vi "进度条.vi"() -> ()   [LabVIEW 2018]
panel:
  in  "诊断结果显示":bool
  out "水平刻度条":dbl(slide) scale=0.0..100.0
  out "进度显示":dbl format="%#.2f%%"
  # "病症诊断进度："
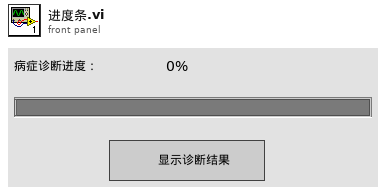
[diagram p1: front panel]
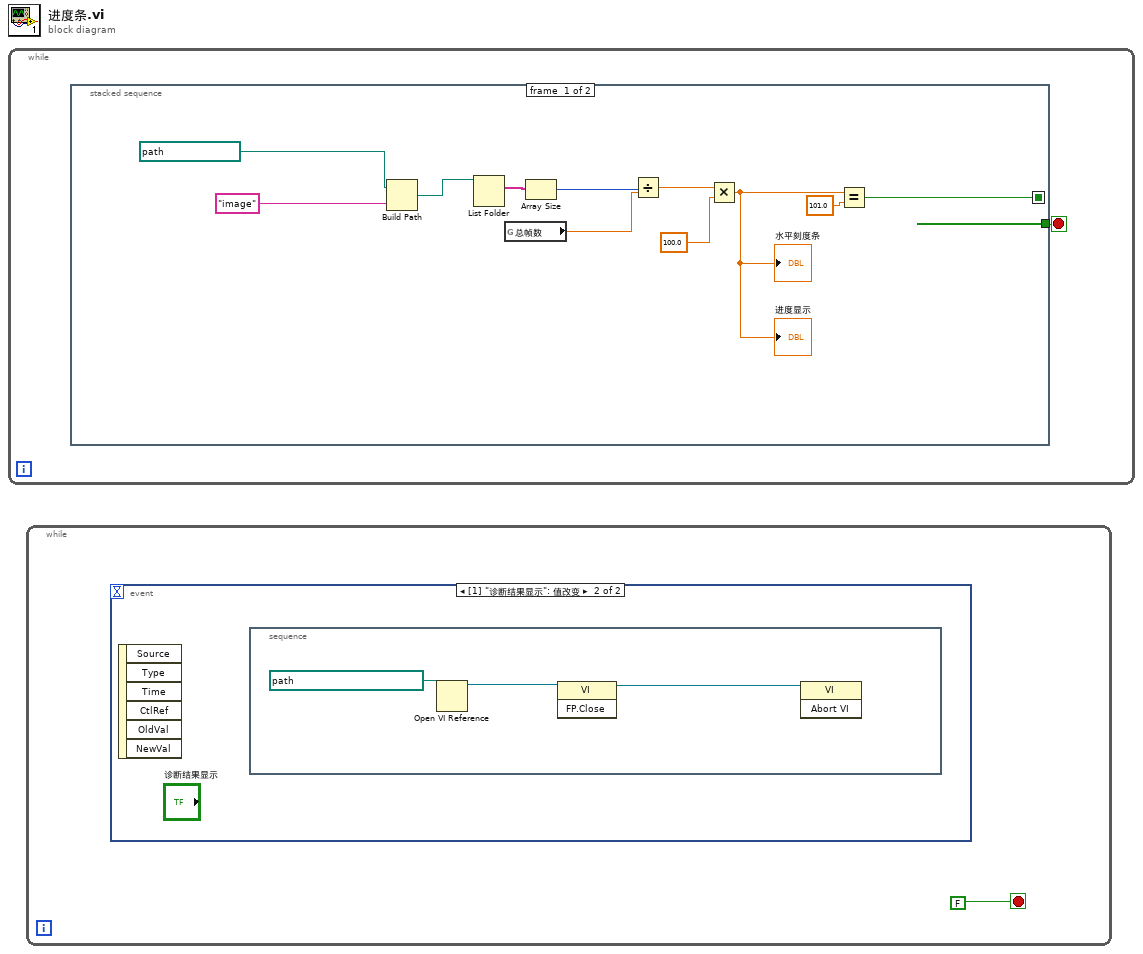
[diagram p0: block diagram]
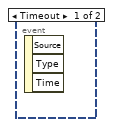
[diagram p2: hidden frame]
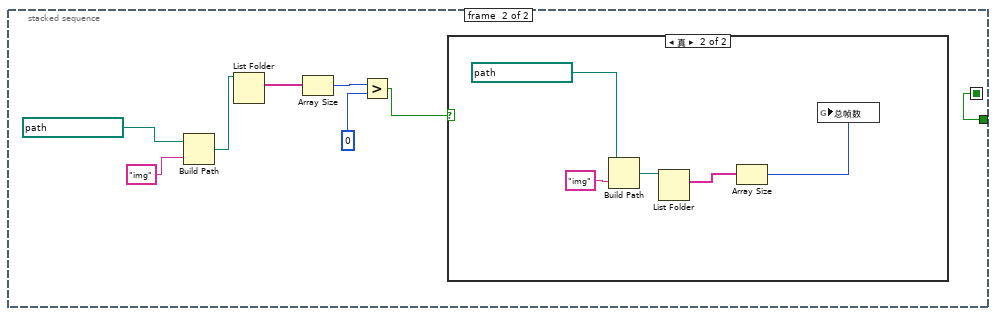
[diagram p3: hidden frame]
diagram:
  n1 = while {
    stop <- w1 stop-if-true
    n2 = stacked-sequence {
      seq-local: [w5 _] -> [_ w20]
      tunnel: [_ w20] -> w1
      frame #0 {
        n3 = Build Path(base path=path "E:/登陆系统重写", name or relative path="image" ("名称或相对路径")) -> (appended path=w10:path)
        n4 = List Folder(path=w10) -> (filenames=w11:string[])  [unwired: 3 in, 3 out]
        n5 = global read "全局变量.vi" "总帧数"() -> (w4:dbl)
        n6 = Array Size(array=w11) -> (size(s)=w3:i32)
        n7 = Divide(x=w3, y=w4) -> (x/y=w8:dbl)
        n8 = Multiply(x=w8, y=100.0) -> (x*y=w7:dbl)
        "水平刻度条" <- w7
        "进度显示" <- w7
        n9 = Equal?(x=w7, y=101.0) -> (x = y?=w5:bool)
      }
      frame #1 {
        n10 = Build Path ("创建路径")(base path=path "E:/登陆系统重写", name or relative path="img" ("名称或相对路径")) -> (appended path=w18:path)
        n11 = List Folder(path=w18) -> (filenames=w17:string[])  [unwired: 3 in, 3 out]
        n12 = Array Size(array=w17) -> (size(s)=w16:i32)
        n13 = Greater?(x=w16, y=0) -> (0:w14:bool)
        n14 = case shown="真" w14 {
          frame False {
          }
          frame True {
            n15 = Build Path(base path=path "E:/登陆系统重写", name or relative path="img" ("名称或相对路径")) -> (appended path=w24:path)
            n16 = List Folder(path=w24) -> (filenames=w25:string[])  [unwired: 3 in, 3 out]
            n17 = Array Size(array=w25) -> (size(s)=w21:i32)
            n18 = global write "全局变量.vi" "总帧数"(w21) -> ()
          }
        }
      }
    }
  }
  n19 = while {
    stop <- FALSE stop-if-true
    n20 = event shown="[1] \"诊断结果显示\": 值改变" {
      selector: _ -> [_ _]
      dyn-events: _ -> [_ _]
      timeout: _ -> [_ _]
      event Timeout {
        n21 = event-data() -> ()  [unwired: 1 in, 3 out]
      }
      event "诊断结果显示": Value Change {
        n22 = event-data() -> ()  [unwired: 1 in, 6 out]
        n23 = stacked-sequence {
          frame #0 {
            n24 = Open VI Reference(vi path=path "E:/登陆系统重写/进度条.vi") -> (vi reference=w29:refnum<vi>)  [unwired: 5 in, 1 out]
            n25 = invoke class="VI" method="FP.Close"(reference=w29) -> (reference out=w28:refnum<vi>)  [unwired: 2 in, 2 out]
            n26 = invoke class="VI" method="Abort VI"(reference=w28) -> ()  [unwired: 2 in, 3 out]
          }
        }
      }
    }
  }
